vi "Validate JWT.vi"(8 "error in (no error)":errorcluster, 9 "Issuer URI path (component)":string, 10 "Client ID":string, 11 "JSONWebToken in":refnum<class "JSONWebToken.lvclass">) -> (0 "error out":errorcluster, 1 "Valid JWT?":bool, 2 "date/time claims":T1, 3 "JSONWebToken out":refnum<class "JSONWebToken.lvclass">)   [LabVIEW 2017, in "JSONWebToken.lvclass"]
doc: "https://openid.net/specs/openid-connect-basic-1_0.html#IDTokenValidation\n\nThe Client MUST validate the ID Token in the Token Response. To do this, the Client can split the ID Token at the period (\".\") characters, take the second segment, and base64url decode it to obtain a JSON object containing the ID Token Claims, which MUST be validated as follows:\n\nThe Issuer Identifier for the OpenID Provider (which is typically obtained during Discovery) MUST exactly match the value of the iss (issuer) Claim.\n\nThe Client MUST validate that the aud (audience) Claim contains its client_id value registered at the Issuer identified by the iss (issuer) Claim as an audience. The ID Token MUST be rejected if the ID Token does not list the Client as a valid audience, or if it contains additional audiences not trusted by the Client.\n\nThe current time MUST be before the time represented by the exp Claim (possibly allowing for some small leeway to account for clock skew).\n\nThe iat Claim can be used to reject tokens that were issued too far away from the current time, limiting the amount of time that nonces need to be stored to prevent attacks. The acceptable range is Client specific.\nIf the acr Claim was requested, the Client SHOULD check that the asserted Claim Value is appropriate. The meaning and processing of acr Claim Values is out of scope for this specification.\n\nWhen a max_age request is made, the Client SHOULD check the auth_time Claim value and request re-authentication if it determines too much time has elapsed since the last End-User authentication."
uses:
  JSONWebToken.lvclass
  JSONWebToken.lvclass/JSONWebToken.ctl
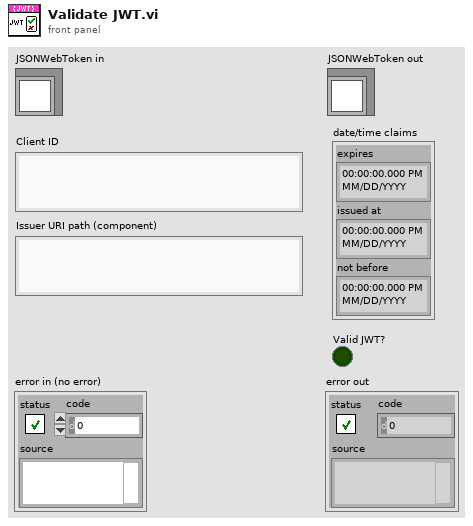
[diagram p1: front panel]
types:
  T1 = cluster{"expires":timestamp, "issued at":timestamp, "not before":timestamp}
  T2 = typedef "header.ctl" = cluster{"alg":string, "jku":string, "jwk":string, "kid":string, "x5u":string, "x5c":string, "x5t":string, "x5t#S256":string, "typ":string, "cty":string, "crit":string, "enc":string}
  T3 = typedef "JSONWebToken.lvclass/JWT registered Claims -- cluster.ctl" = cluster{"iss":string, "sub":string, "aud":string, "exp":i32, "iat":i32, "nbf":i32, "jti":string, "nonce":string, "at_hash":string, "acr":string, "amr":string}
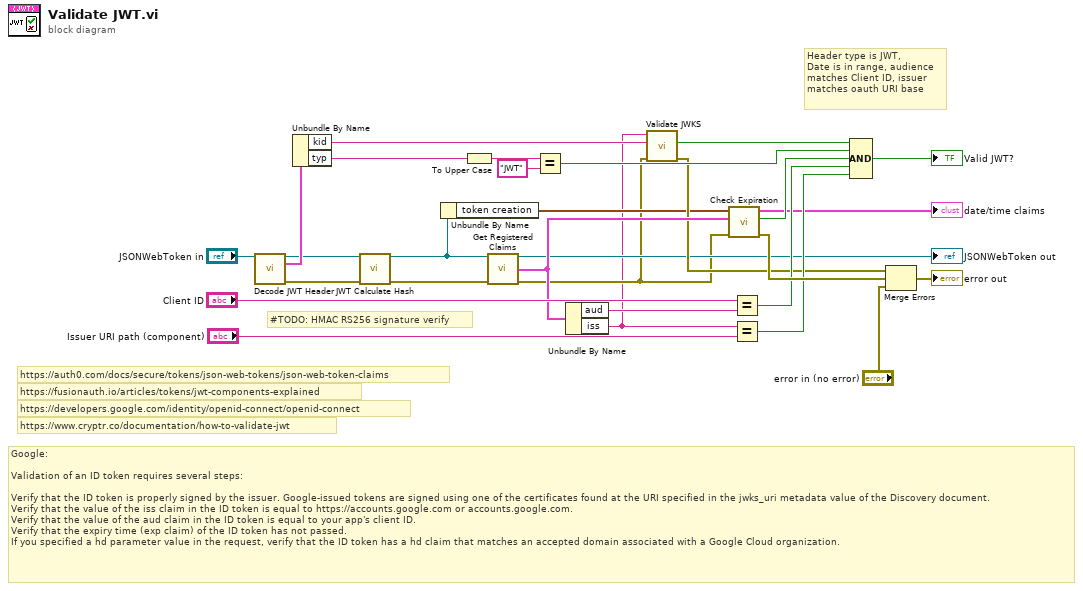
[diagram p0: block diagram]
diagram:
  # "Header type is JWT,\nDate is in range, audience \nmatches Client ID, issuer\nmatches oauth URI base"
  # "#TODO: HMAC RS256 signature verify"
  # "https://developers.google.com/identity/openid-connect/openid-connect"
  # "Google:\n\nValidation of an ID token requires several steps:\n\nVerify that the ID token is properly signed by the issuer. Google-issued tokens are signed using one of the certificates found at the URI specified in the jwks_uri metadata value of the Discovery document.\nVerify that the value of the iss claim in the ID token is equal to https://accounts.google.com or accounts.google.com.\nVerify that the value of the aud claim in the ID token is equal to your app's client ID.\nVerify that the expiry time (exp claim) of the ID token has not passed.\nIf you specified a hd parameter value in the request, verify that the ID token has a hd claim that matches an accepted domain associated with a Google Cloud organization."
  # "https://fusionauth.io/articles/tokens/jwt-components-explained"
  # "https://auth0.com/docs/secure/tokens/json-web-tokens/json-web-token-claims"
  # "https://www.cryptr.co/documentation/how-to-validate-jwt"
  n1 = call "Decode JWT Header.vi"("JSONWebToken in"="JSONWebToken in") -> ("JSONWebToken out"=w4:refnum<class "JSONWebToken.lvclass">, "JWT header"=w21:T2, "error out"=w6:errorcluster)  [unwired: 11 in, 1 out]
  n2 = Unbundle By Name(w21) -> ("kid"=w19:string, "typ"=w20:string)
  n3 = call "JWT Calculate Hash.vi"("JSONWebToken in"=w4, "error in (no error)"=w6) -> ("JSONWebToken out"=w3:refnum<class "JSONWebToken.lvclass">, "error out"=w5:errorcluster)  [unwired: 11 in, 1 out]
  n4 = Unbundle By Name(w3) -> ("token creation"=w7:timestamp)
  n5 = To Upper Case(1:w20) -> (0:w25:string)
  n6 = call "Get Registered Claims.vi"("JSONWebToken in"=w3, "error in (no error)"=w5) -> ("JSONWebToken out"=→"JSONWebToken out":refnum<class "JSONWebToken.lvclass">, "registered claims"=w16:T3, "error out"=w2:errorcluster)  [unwired: 10 in, 1 out]
  n7 = Equal?(x=w25, y="JWT") -> (x = y?=w22:bool)
  n8 = Unbundle By Name(w16) -> ("aud"=w24:string, "iss"=w1:string)
  n9 = call "Validate JWKS.vi"("error in (no error)"=w2, "kid"=w19, "Issuer URI path"=w1) -> ("error out"=w11:errorcluster, "kid found?"=w17:bool)  [unwired: 4 in, 3 out]
  n10 = call "Check Expiration.vi"("error in (no error)"=w2, "registered claims"=w16, "token creation"=w7) -> ("error out"=w29:errorcluster, "datetime valid"=w10:bool, "date/time claims"=→"date/time claims":T1)  [unwired: 6 in]
  n11 = Equal?(x="Client ID", y=w24) -> (x = y?=w23:bool)
  n12 = Equal?(x=w1, y="Issuer URI path (component)") -> (x = y?=w18:bool)
  n13 = Compound Arithmetic op=AND(w17, w22, w10, w23, w18) -> (→"Valid JWT?":bool)
  n14 = Merge Errors(w11, w29, "error in (no error)") -> (→"error out":errorcluster)
